vi "Handix Interface.vi"() -> ()   [LabVIEW 2015]
uses:
  CRD/Data/tCRD Data.lvclass
  Reusable/Xctls/Configurable Buffer/Configurable Buffer.xctl
  <vilib>/Utility/miscctls.llb/LVPositionTypeDef.ctl
  <vilib>/event_ctls.llb/eventvkey.ctl
  Devices/Alicat/Session Based/Data/MC/MC Data.lvclass
  Reusable/General/Math Utilities.lvlib
  <vilib>/Analysis/NI_AALBase.lvlib
  <vilib>/Analysis/1siggen.llb/Ramp Pattern by Delta.vi
  Reusable/CRDS/Data/Cell/CRDS Cell Data.lvclass
  Devices/Airmar/Data/Airmar Data.lvclass
  FPGA/Rate.ctl
  Reusable/CRDS/Data/Cell/extparam.ctl
panel:
  in  "writeTaus":bool
  out "filtLastSw":timestamp caption="Last Zero" format="%<%H:%M:%S%2u\n%m/%d>T"
  in  "tSwitch":dbl caption="Next Switch (s)"
  in  "newFile":bool
  in  "restart":bool
  in  "SyncTime":bool
  out "Zeroing?":bool
  in  "writeRDs":bool
  in  "mainTab":enum32{"Main", "Control", "Auxilary"}(tab)
  out "rd":dbl[][](graph)
  out "tau (us)":sgl
  out "Data In":sgl(graph)
  out "eRD":dbl[](graph)
  in  "Invert?":bool
  out "Drive Space (Mb)":u32
  in  "Qpurge (lpm)":cluster{"Sample":sgl, "Zero":sgl} {"Zero" min=0 step=0.01 format="%.2g"; "Sample" min=0 step=0.01 format="%.2g"}
  out "Alicat Data":T1
  in  "Laser Off (us)":u32=16
  in  "# to Coadd":u8=16 min=1 max=50 step=1
  in  "Bank 3":bool
  in  "Bank 2":bool
  in  "Bank 1":bool
  in  "Rate":T2=10 items=["1 MHz"=20, "2 MHz"=10, "2.5 MHz"=8, "5 MHz"=4, "10 MHz"=2, "20MHz"=1]
  in  "Sample Time (us)":u16=100
  in  "Delay (us)":u16=16
  in  "Frequency (Hz)":dbl
  in  "cycle?":bool
  in  "Sample (s)":dbl
  in  "Zero (s)":dbl
  in  "Servo Position (deg)":cluster{u32, u32}(slide)={806, 2337} scale=500.0..2500.0
  in  "Lock":bool=TRUE
  in  "Zero State":bool
  out "vData":cluster{"RH (%)":sgl, "T deg(C)":sgl} caption="Vaisala Data" {"T deg(C)" format="%6.2f"; "RH (%)" format="%6.2f"}
  out "Path":path
  out "File Size":u32
  out "extParam":T3={"Tau"=nan, "Tau0cor"=nan, "ext"=nan, "extCorr"=nan, "stdevTau"=nan, "eTau"=nan, "taucorr"=nan, "Tau0"=nan, "max"=nan} caption="Extinction Parameters" {"Tau0" format="%#.2f"; "taucorr" format="%#.2f"; "eTau" format="%#.2f"; "stdevTau" format="%#.2f"; "extCorr" format="%.2f"; "ext" format="%#.2f"; "Tau0cor" format="%#.2f"; "Tau" format="%#.2f"}
  out "Tv":cluster{"Val":dbl[], "time":timestamp}(xcontrol)
  out "RHv":cluster{"Val":dbl[], "time":timestamp}(xcontrol)
  out "Anemometer":cluster{"Val":dbl[], "time":timestamp}(xcontrol)
  out "Version":string
  in  "Save":bool
  out "time":timestamp format="%<%H:%M:%S%2u>T"
  # "CRD Zero"
  # "OPEN PATH DATA"
  # "CONTROL"
  # "Open Path CRD Control"
  # "Laser/Sample Control"
  # "Servo"
  # "Fan Control"
  # "AUXILARY DATA"
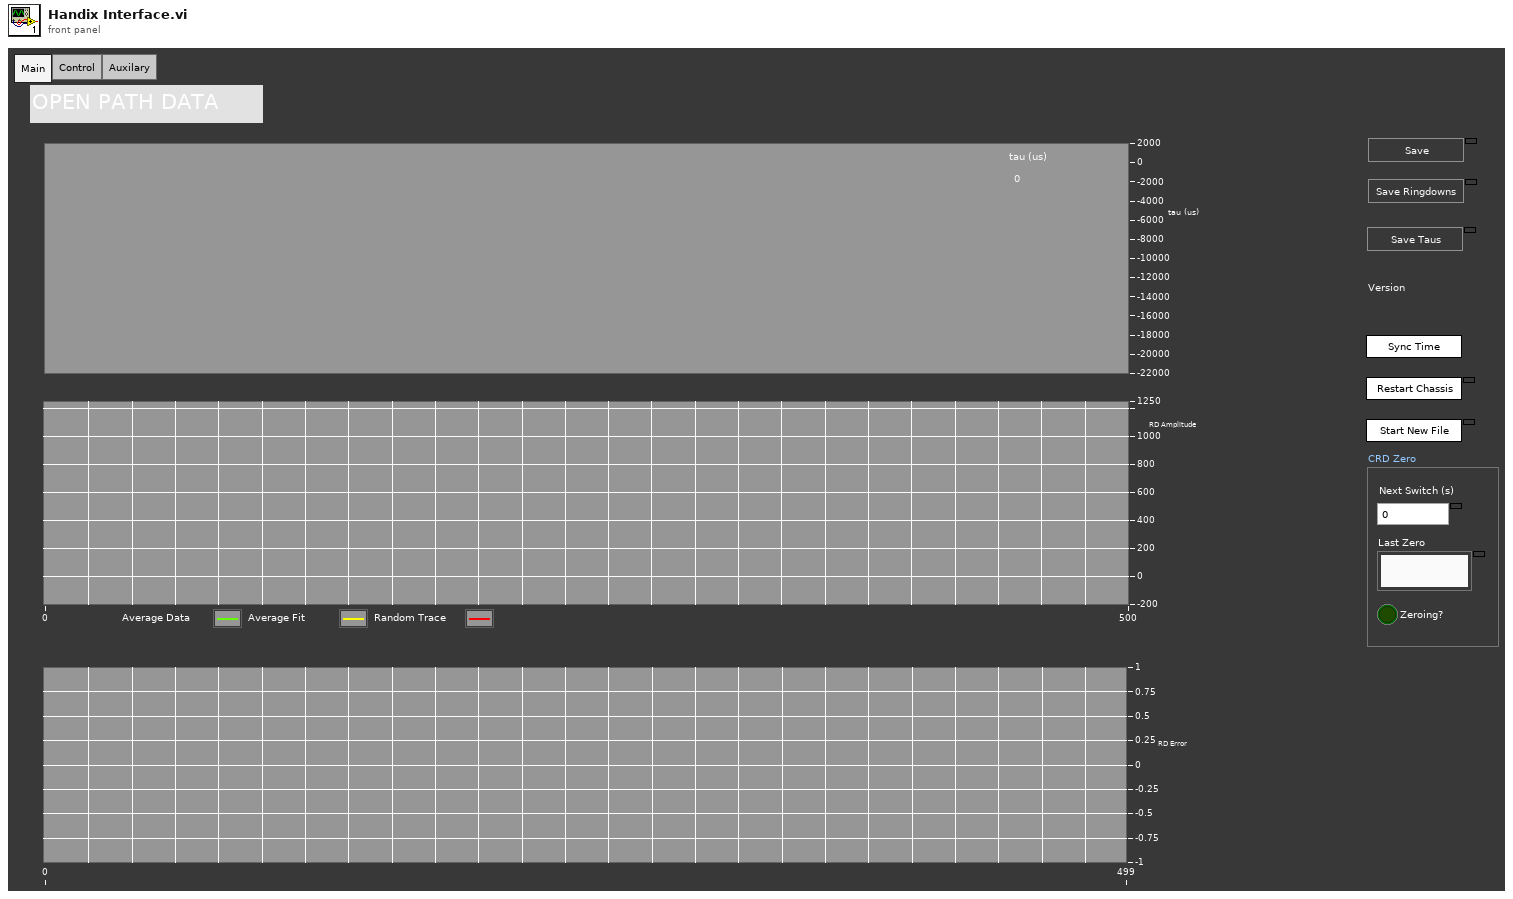
[diagram p1: front panel]
types:
  T1 = cluster{"P (mb)":dbl, "T (degC)":dbl, "Q (lpm)":dbl, "Q (slpm)":dbl, "Qsp":dbl}
  T2 = typedef "Rate.ctl" = u8
  T3 = typedef "extparam.ctl" = cluster{"Tau":sgl, "Tau0cor":sgl, "ext":sgl, "extCorr":sgl, "stdevTau":sgl, "eTau":sgl, "taucorr":sgl, "Tau0":sgl, "max":sgl}
  T4 = enum32{"Invalid", "Standard", "Closed", "Hidden", "Minimized", "Maximized"}
  T5 = typedef "LVPositionTypeDef.ctl" = cluster{"Left":i32, "Top":i32}
  T6 = typedef "eventvkey.ctl" = enum16{"ASCII", "Enter", "Return", "Shift", "Ctrl", "Alt", "Cmd", "Opt", "Caps", "NumLock", "Clear", "Break", "Up", "Down", "Left", "Right", "Insert", "Delete", "Home", "End", "PageUp", "PageDown", "Escape", "Help", "Pause", "ScrollLock", "F1", "F2", "F3", "F4", "F5", "F6", "F7", "F8", "F9", "F10", "F11", "F12", "F13", "F14", "F15", "F16", "F17", "F18", "F19", "F20", "F21", "F22", "F23", "F24", "Play", "VolumeUp", "VolumeDown", "Mute", "Two Byte Char"}
  T7 = enum8{"Enabled", "Disabled", "Disabled and Grayed Out"}
  T8 = cluster{"Barometric Pressure":dbl, "Temperature":dbl, "Relative Humidity":dbl, "Dew Point":dbl, "True Wind Direction":dbl, "Magnetic Wind Direction":dbl, "Wind Speed":dbl}
  T9 = cluster{"Accessors:P":sgl, "Accessors:T":sgl, "Accessors:Q":sgl, "Accessors:Q0":sgl, "Accessors:Qsp":sgl}
  T10 = cluster{"Array of Single[0]":sgl, "Array of Single[1]":sgl}
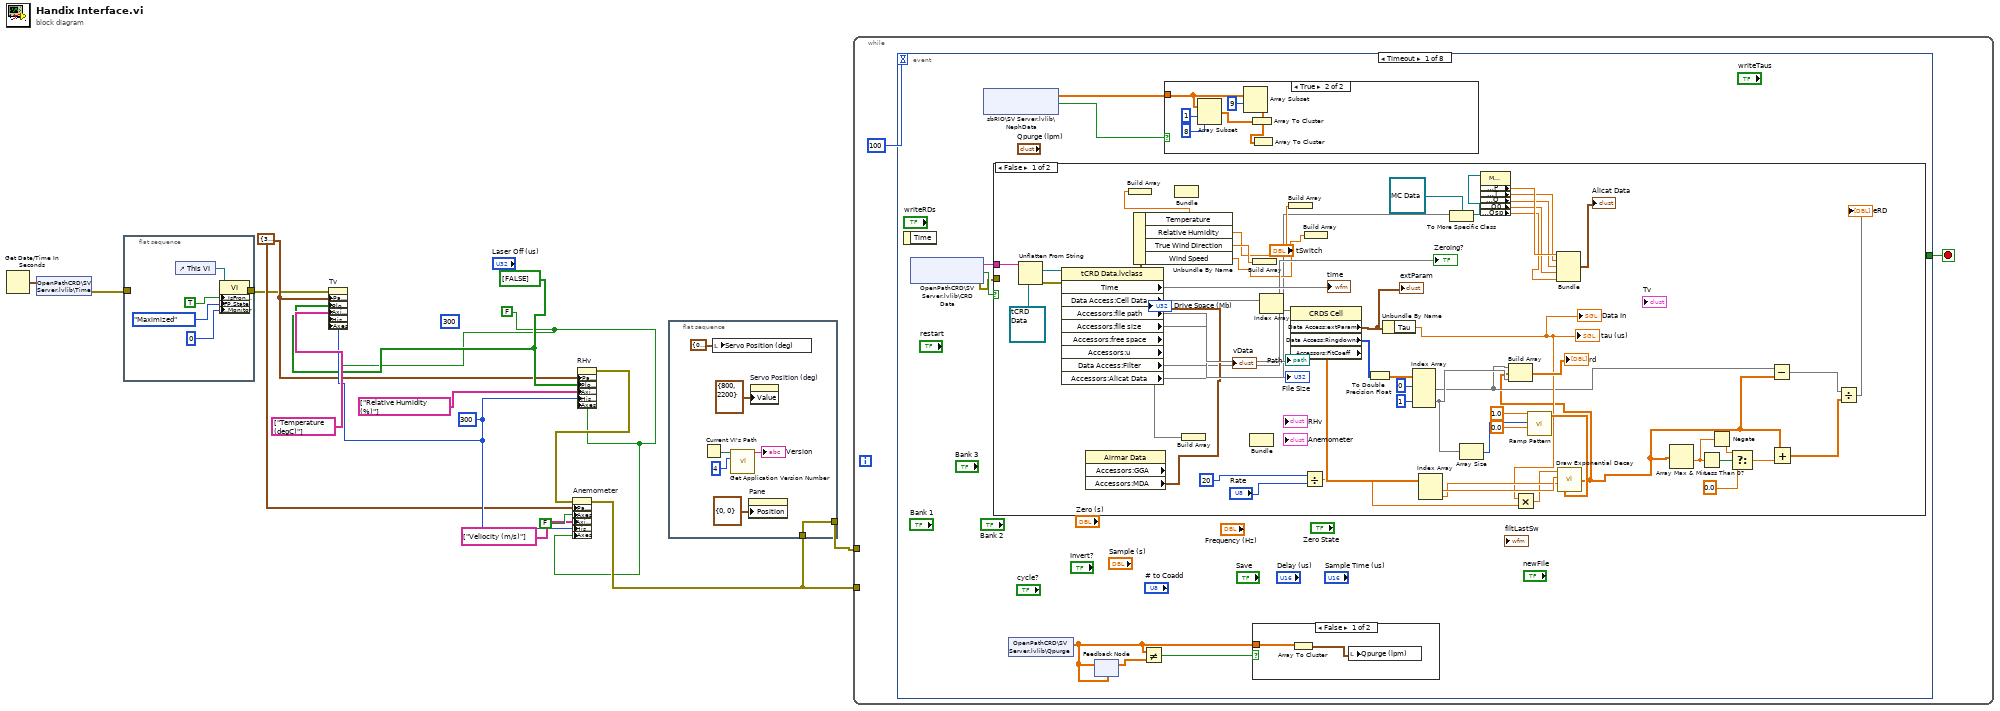
[diagram p0: block diagram]
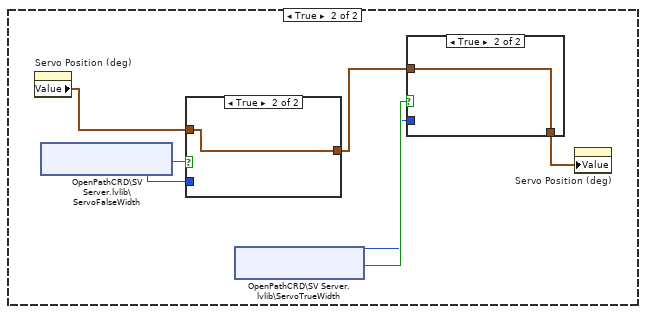
[diagram p4: hidden frame]
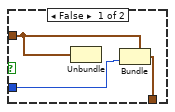
[diagram p5: hidden frame]
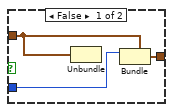
[diagram p6: hidden frame]
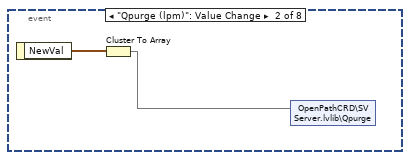
[diagram p7: hidden frame]
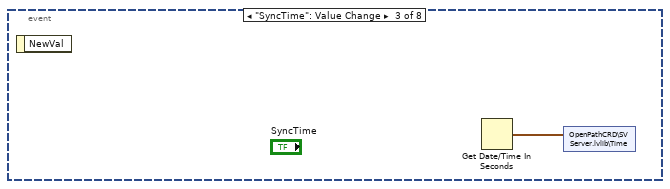
[diagram p8: hidden frame]
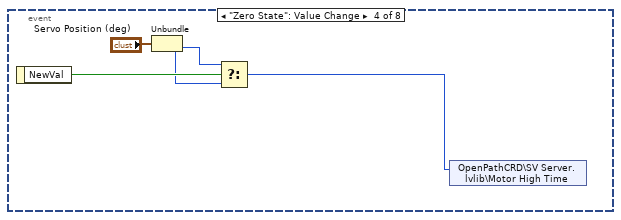
[diagram p9: hidden frame]
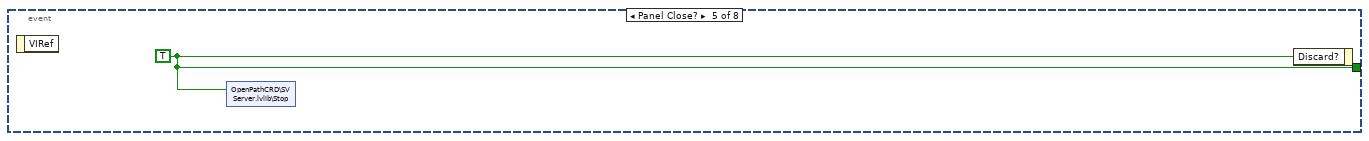
[diagram p10: hidden frame]
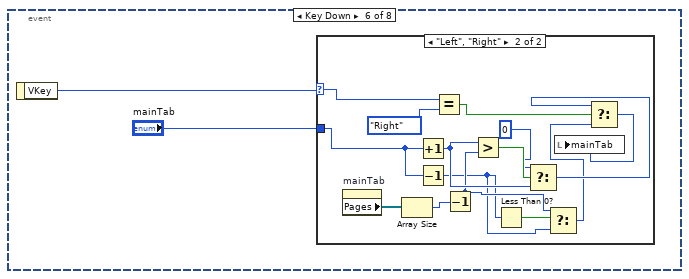
[diagram p11: hidden frame]
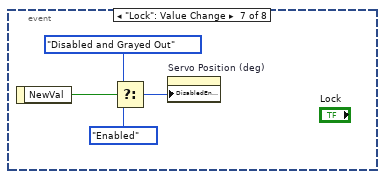
[diagram p13: hidden frame]
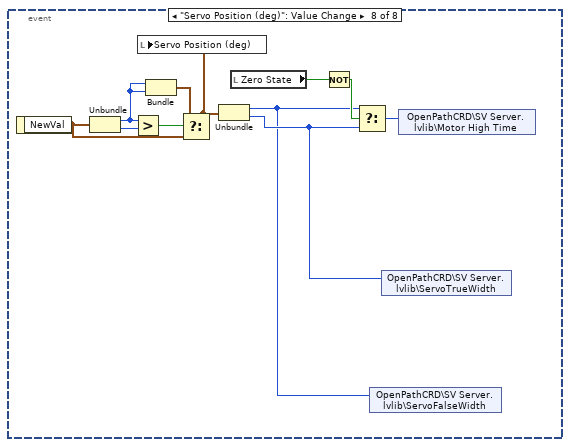
[diagram p14: hidden frame]
diagram:
  w5 = FALSE ("Two Axes?")
  w4 = cluster{"Height":i16, "Width":i16} {"Height"=325, "Width"=525} ("Panel Size")
  w6 = bool[] [FALSE] ("Plot Second Axis?")
  (unwired) 300 ("History")
  w7 = 300 ("History")
  n1 = Get Date/Time In Seconds() -> (seconds since 1Jan1904=w2:timestamp)
  n2 = shared-variable "OpenPathCRD\\SV Server.lvlib\\Time"(w2) -> (error out=w1:errorcluster)  [unwired: 1 in]
  n3 = flat-sequence {
    tunnel: [w15] -> w3
    tunnel: w1 -> [_]
    frame #0 {
      n4 = control-ref of="This VI"() -> (w19:refnum<vi>)
      n5 = property class="VI"(reference=w19, "Front Panel.IsFrontmost"=TRUE ("Front Panel Window:Is Frontmost"), "FP.State"=T4."Maximized" ("Front Panel Window:State"), "FP.Monitor"=u16 0 ("Front Panel Window:Monitor")) -> (error out=w15:errorcluster)  [unwired: 1 in, 1 out]
    }
  }
  n6 = property on="Tv"(error in=w3, "Panel Size"=w4, "Plot Second Axis?"=w6, "Axis Name"=string[] ["Temperature (degC)"], "History (2)"=w7, "Axes"=w5) -> ()  [unwired: 1 in, 2 out]
  n7 = property on="RHv"("Panel Size"=w4, "Plot Second Axis?"=w6, "Axis Name"=string[] ["Relative Humidity (%)"], "History (2)"=w7, "Axes"=w5) -> (error out=w14:errorcluster)  [unwired: 2 in, 1 out]
  n8 = property on="Anemometer"(error in=w14, "Panel Size"=w4, "Axes"=FALSE ("Two Axes?"), "Axis Name"=string[] ["Veliocity (m/s)"], "History (2)"=w7, "Axes"=w5) -> (error out=w9:errorcluster)  [unwired: 1 in, 1 out]
  n9 = flat-sequence {
    tunnel: [w20] -> w10
    tunnel: w9 -> [w20]
    frame #0 {
      n10 = Current VI's Path() -> (path=w23:path)
      n11 = local write "Servo Position (deg)"(cluster{dbl, dbl} {0.0, 90.0} ("Servo Position (deg)")) -> ()
      n12 = call "Get Application Version Number.vi"("Number to Strip"=4, "Initial Path"=w23) -> ("Version"=→"Version":string)  [unwired: 8 in, 1 out]
      n13 = property on="Pane" class="Pane"("Position"=T5 {"Left"=0, "Top"=0}) -> ()  [unwired: 2 in, 2 out]
      n14 = property on="Servo Position (deg)" class="Slide (strict)"("Value"=cluster{u32, u32} {800, 2200} ("Servo Position (deg)")) -> ()  [unwired: 2 in, 2 out]
    }
  }
  n15 = while {
    tunnel: w9 -> [_]
    tunnel: w10 -> [_]
    stop <- w28 stop-if-true
    n16 = event shown="[0] Timeout" {
      selector: _ -> [_ _ _ _ _ _ _ _]
      dyn-events: _ -> [_ _ _ _ _ _ _ _]
      timeout: 100 -> [_ _ _ _ _ _ _ _]
      tunnel: [_ _ _ _ w122 _ _ _] -> w28
      event Timeout {
        n17 = event-data() -> ()  [unwired: 1 in, 1 out]
        n18 = shared-variable "OpenPathCRD\\SV Server.lvlib\\CRD Data"() -> (w36:string, error out=w29:errorcluster, w35:bool)  [unwired: 2 in]
        n19 = shared-variable "sbRIO\\SV Server.lvlib\\NephData"() -> (w33:dbl[], w34:bool)  [unwired: 2 in, 1 out]
        n20 = case shown="False" w35 {
          tunnel: w36 -> [w98 _]
          tunnel: w29 -> [_ _]
          frame False {
            n21 = Unflatten From String(type=refnum<class "tCRD Data.lvclass"> refnum ("tCRD Data"), binary string=w98) -> (value=w97:refnum<class "tCRD Data.lvclass">, error out=w96:errorcluster)  [unwired: 3 in, 1 out]
            n22 = property class="tCRD Data.lvclass" props=["Time", "Data Access:Cell Data", "Accessors:file path", "Accessors:file size", "Accessors:free space", "Accessors:u", "Data Access:Filter", "Accessors:Alicat Data"](reference=w97, error in=w96) -> ("Time"=→"time", "Data Access:Cell Data"=w95, "Accessors:file path"=→"Path", "Accessors:file size"=→"File Size", "Accessors:u"=w85, "Data Access:Filter"=→"Zeroing?", "Accessors:Alicat Data"=w77)  [unwired: 3 out]
            n23 = property class="Airmar Data" props=["Accessors:GGA", "Accessors:MDA"]() -> ("Accessors:MDA"=w84:T8)  [unwired: 2 in, 3 out]
            n24 = Unbundle By Name(w84) -> ("Temperature"=w80:dbl, "Relative Humidity"=w82:dbl, "True Wind Direction"=w83:dbl, "Wind Speed"=w79:dbl)
            n25 = Build Array(w80) -> ()  [unwired: 1 out]
            n26 = Bundle() -> ()  [unwired: 3 in, 1 out]
            n27 = Build Array(w85) -> ()  [unwired: 1 out]
            n28 = Bundle() -> ()  [unwired: 3 in, 1 out]
            n29 = Build Array(w83) -> ()  [unwired: 1 out]
            n30 = Index Array(array=w95) -> (element=w94)  [unwired: 1 in]
            n31 = Build Array(w82) -> ()  [unwired: 1 out]
            n32 = property class="CRDS Cell"(reference=w94) -> ("Data Access:extParam"=w69:T3, "Data Access:Ringdowns"=w88:i16[][], "Accessors:FitCoeff"=w68:dbl[])  [unwired: 1 in, 2 out]
            "extParam" <- w69
            n33 = Divide(x=20, y="Rate") -> (x/y=w56:dbl)
            n34 = Build Array(w79) -> ()  [unwired: 1 out]
            n35 = To Double Precision Float(number=w88) -> (double precision float=w87:dbl[][])
            n36 = Unbundle By Name(w69) -> ("Tau"=w57:sgl)
            "Data In" <- w57
            "tau (us)" <- w57
            n37 = Index Array(array=w87, index (row) #1=0 ("index (row)"), index (row) #2=1 ("index (row)")) -> (element #1=w49:dbl[], element #2=w63:dbl[])  [unwired: 2 in]
            n38 = Index Array(array=w68) -> (element #1=w67:dbl, element #2=w66:dbl)  [unwired: 2 in]
            n39 = To More Specific Class(target class=refnum<class "MC Data.lvclass"> refnum ("MC Data"), reference=w77) -> (specific class reference=w76:refnum<class "MC Data.lvclass">)  [unwired: 1 in, 1 out]
            n40 = Array Size(array=w63) -> (size(s)=w62:i32)
            n41 = property class="MC Data"(reference=w76) -> ("Accessors:P"=w75:sgl, "Accessors:T"=w74:sgl, "Accessors:Q"=w73:sgl, "Accessors:Q0"=w72:sgl, "Accessors:Qsp"=w71:sgl)  [unwired: 1 in, 2 out]
            n42 = Multiply(x=w57, y=w56) -> (x*y=w55:dbl)
            n43 = call-poly <vilib>:"Ramp Pattern.vi"("start"=0.0, "end"=w62, "delta"=1.0) -> ("Ramp Pattern"=w65:dbl[])  [unwired: 6 in, 2 out]
            n44 = Bundle("Accessors:P"=w75, "Accessors:T"=w74, "Accessors:Q"=w73, "Accessors:Q0"=w72, "Accessors:Qsp"=w71) -> (→"Alicat Data":T9)  [unwired: 1 in]
            n45 = call "Draw Exponential Decay.vi"("time"=w65, "B"=w66, "A"=w67, "tau"=w55) -> ("ExponentialOut"=w45:dbl[])
            n46 = Build Array(w49, w45, w63) -> (→"rd":dbl[][])
            n47 = Array Max & Min(array=w45) -> (min value=w47:dbl)  [unwired: 3 out]
            n48 = Less Than 0?(x=w47) -> (x < 0?=w54:bool)
            n49 = Negate(x=w47) -> (-x=w46:dbl)
            n50 = Select(t=w46, s=w54, f=0.0) -> (s? t:f=w48:dbl)
            n51 = Subtract(x=w49, y=w45) -> (x-y=w52:dbl[])
            n52 = Add(x=w45, y=w48) -> (x+y=w50:dbl[])
            n53 = Divide(x=w52, y=w50) -> (x/y=→"eRD":dbl[])
          }
          frame True {
            n54 = property on="Servo Position (deg)" class="Slide (strict)"() -> ("Value"=w104:cluster{u32, u32})  [unwired: 2 in, 2 out]
            n55 = shared-variable "OpenPathCRD\\SV Server.lvlib\\ServoFalseWidth"() -> (w103:u32, w105:bool)  [unwired: 2 in, 1 out]
            n56 = case shown="True" w105 {
              tunnel: w104 -> [w112 w113]
              tunnel: w103 -> [w111 _]
              tunnel: [w110 w113] -> w102
              frame False {
                n57 = Unbundle(w112) -> ()  [unwired: 2 out]
                n58 = Bundle(cluster=w112, w111) -> (w110:cluster{u32, u32})  [unwired: 1 in]
              }
              frame True {
              }
            }
            n59 = shared-variable "OpenPathCRD\\SV Server.lvlib\\ServoTrueWidth"() -> (w100:u32, w101:bool)  [unwired: 2 in, 1 out]
            n60 = case shown="True" w101 {
              tunnel: w102 -> [w108 w109]
              tunnel: w100 -> [w107 _]
              tunnel: [w106 w109] -> w99
              frame False {
                n61 = Unbundle(w108) -> ()  [unwired: 2 out]
                n62 = Bundle(cluster=w108, w107) -> (w106:cluster{u32, u32})  [unwired: 1 in]
              }
              frame True {
              }
            }
            n63 = property on="Servo Position (deg)" class="Slide (strict)"("Value"=w99) -> ()  [unwired: 2 in, 2 out]
          }
        }
        n64 = shared-variable "OpenPathCRD\\SV Server.lvlib\\Qpurge"() -> (w30:sgl[])  [unwired: 1 in, 1 out]
        n65 = feedback-in #1(w30) -> ()
        n66 = feedback #1(w30) -> (w32:sgl[])
        n67 = Not Equal?(x=w30, y=w32) -> (x != y?=w31:bool)
        n68 = case shown="True" w34 {
          tunnel: w33 -> [_ w41]
          frame False {
          }
          frame True {
            n69 = Array Subset(array=w41, index=1, length=8) -> (w42:dbl[])
            n70 = Array Subset(array=w41, index=9) -> (w39:dbl[])  [unwired: 1 in]
            n71 = Array To Cluster(array=w42) -> ()  [unwired: 1 out]
            n72 = Array To Cluster(array=w39) -> ()  [unwired: 1 out]
          }
        }
        n73 = case shown="False" w31 {
          tunnel: w30 -> [w38 _]
          frame False {
            n74 = Array To Cluster(array=w38) -> (cluster=w37:T10)
            n75 = local write "Qpurge (lpm)"(w37) -> ()
          }
          frame True {
          }
        }
      }
      event "Qpurge (lpm)": Value Change {
        n76 = event-data() -> ("NewVal"=w115:cluster{"Sample":sgl, "Zero":sgl})  [unwired: 1 in]
        n77 = Cluster To Array(cluster=w115) -> (array=w114:sgl[])
        n78 = shared-variable "OpenPathCRD\\SV Server.lvlib\\Qpurge"(w114) -> ()  [unwired: 1 in, 1 out]
      }
      event "SyncTime": Value Change {
        n79 = event-data() -> ()  [unwired: 1 in, 1 out]
        n80 = Get Date/Time In Seconds() -> (seconds since 1Jan1904=w116:timestamp)
        n81 = shared-variable "OpenPathCRD\\SV Server.lvlib\\Time"(w116) -> ()  [unwired: 1 in, 1 out]
      }
      event "Zero State": Value Change {
        n82 = event-data() -> ("NewVal"=w121:bool)  [unwired: 1 in]
        n83 = Unbundle("Servo Position (deg)") -> (w119:u32, w118:u32)
        n84 = Select(t=w118, s=w121, f=w119) -> (s? t:f=w117:u32)
        n85 = shared-variable "OpenPathCRD\\SV Server.lvlib\\Motor High Time"(w117) -> ()  [unwired: 1 in, 1 out]
      }
      event Panel Close? {
        w122 = TRUE ("Discard?")
        n86 = event-data() -> ()  [unwired: 1 in, 1 out]
        n87 = shared-variable "OpenPathCRD\\SV Server.lvlib\\Stop"(w122) -> ()  [unwired: 1 in, 1 out]
        n88 = event-data("Discard?"=w122) -> ()  [unwired: 1 in, 1 out]
      }
      event Key Down {
        n89 = event-data() -> ("VKey"=w124:T6)  [unwired: 1 in]
        n90 = case shown="\"Left\", \"Right\"" w124 {
          selector: w124 -> [_ w138]
          tunnel: "mainTab" -> [_ w130]
          frame "ASCII", Default {
          }
          frame "Left", "Right" {
            n91 = property on="mainTab" class="TabCtl (strict)"() -> ("Pages"=w139:refnum<vi>[])  [unwired: 2 in, 2 out]
            n92 = Array Size(array=w139) -> (size(s)=w135:i32)
            n93 = Increment(x=w130) -> (x+1=w133:enum32{"Main", "Control", "Auxilary"})
            n94 = Decrement(x=w130) -> (x-1=w127:enum32{"Main", "Control", "Auxilary"})
            n95 = Equal?(x=w138, y=eventvkey."Right") -> (x = y?=w136:bool)
            n96 = Decrement(x=w135) -> (x-1=w128:i32)
            n97 = Greater?(x=w133, y=w128) -> (0:w134:bool)
            n98 = Less Than 0?(x=w127) -> (x < 0?=w129:bool)
            n99 = Select(t=0, s=w134, f=w133) -> (s? t:f=w131:u32)
            n100 = Select(t=w128, s=w129, f=w127) -> (s? t:f=w126:u32)
            n101 = Select(t=w131, s=w136, f=w126) -> (s? t:f=w125:u32)
            n102 = local write "mainTab"(w125) -> ()
          }
        }
      }
      event "Lock": Value Change {
        n103 = event-data() -> ("NewVal"=w143:bool)  [unwired: 1 in]
        n104 = Select(t=T7."Disabled and Grayed Out" ("Disabled"), s=w143, f=T7."Enabled" ("Disabled")) -> (s? t:f=w140:T7)
        n105 = property on="Servo Position (deg)" class="Slide (strict)"("DisabledEnum"=w140) -> ()  [unwired: 2 in, 2 out]
      }
      event "Servo Position (deg)": Value Change {
        n106 = event-data() -> ("NewVal"=w152:cluster{u32, u32})  [unwired: 1 in]
        n107 = Unbundle(w152) -> (w151:u32, w154:u32)
        n108 = Greater?(x=w151, y=w154) -> (0:w153:bool)
        n109 = Bundle(w151, w151) -> (w150:cluster{u32, u32})  [unwired: 1 in]
        n110 = Select(t=w150, s=w153, f=w152) -> (s? t:f=w149:cluster{u32, u32})
        n111 = local write "Servo Position (deg)"(w149) -> ()
        n112 = Unbundle(w149) -> (w144:u32, w145:u32)
        n113 = local read "Zero State"() -> (w147:bool)
        n114 = Not(x=w147) -> (.not. x?=w146:bool)
        n115 = Select(t=w144, s=w146, f=w145) -> (s? t:f=w148:u32)
        n116 = shared-variable "OpenPathCRD\\SV Server.lvlib\\ServoFalseWidth"(w144) -> ()  [unwired: 1 in, 1 out]
        n117 = shared-variable "OpenPathCRD\\SV Server.lvlib\\ServoTrueWidth"(w145) -> ()  [unwired: 1 in, 1 out]
        n118 = shared-variable "OpenPathCRD\\SV Server.lvlib\\Motor High Time"(w148) -> ()  [unwired: 1 in, 1 out]
      }
    }
  }
